vi "Write CAP1208.vi"(8 "error in (no error)":errorcluster, 10 "CAP1208":refnum<class "CAP1208.lvclass">, 11 "LINX-ExplorerHatPro in":refnum<class "LINX-ExplorerHatPro.lvclass">) -> (0 "error out":errorcluster, 3 "LINX-ExplorerHatPro out":refnum<class "LINX-ExplorerHatPro.lvclass">)   [LabVIEW 2020, in "LINX-ExplorerHatPro.lvclass"]
uses:
  LINX-ExplorerHatPro.lvclass
  CAP1208/CAP1208.lvclass
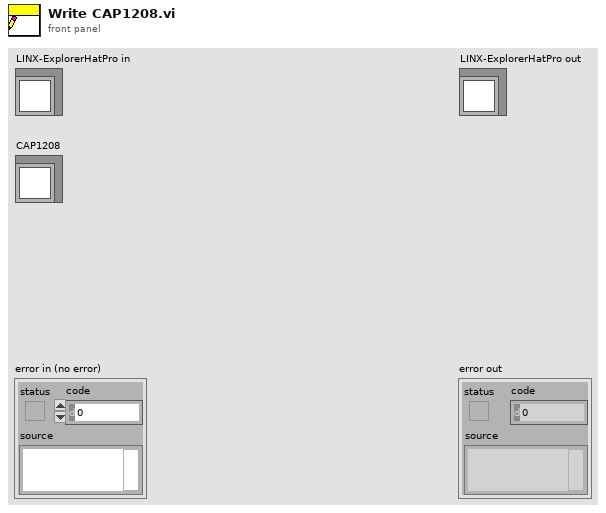
[diagram p1: front panel]
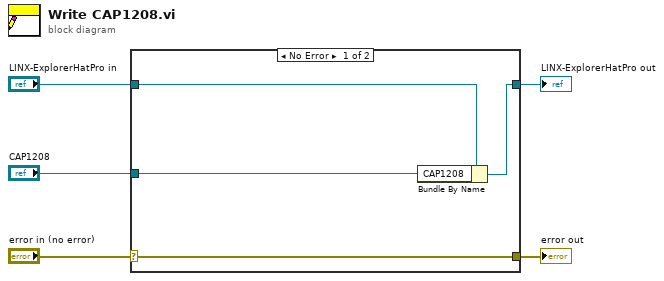
[diagram p0: block diagram]
diagram:
  n1 = case shown="No Error" "error in (no error)" {
    selector: "error in (no error)" -> [w9 w10]
    tunnel: [w9 w10] -> w4
    tunnel: [w7 w11] -> w2
    tunnel: "LINX-ExplorerHatPro in" -> [w8 w11]
    tunnel: "CAP1208" -> [w6 _]
    frame No Error {
      n2 = Bundle By Name(cluster=w8, "CAP1208"=w6) -> (w7:refnum<class "LINX-ExplorerHatPro.lvclass">)
    }
    frame Error {
    }
  }
  "error out" <- w4
  "LINX-ExplorerHatPro out" <- w2
